vi "LVClass_WavefrontCorrector get all WFC parameter values.vi"(0 "WavefrontCorrector in":refnum<class "WavefrontCorrector.lvclass">, 11 "error in (no error)":errorcluster) -> (4 "WavefrontCorrector out":refnum<class "WavefrontCorrector.lvclass">, 6 "AllWFCParametersValues":T1[](array[typedef]), 15 "error out":errorcluster)   [LabVIEW 2020, in "WavefrontCorrector.lvclass"]
doc: "Description:\nGet current actuators positions.\n\nParameters:\nclass corrector WavefrontCorrector object adress.\nfloat position Array containing the actuators positions.\nError error_in [in] Error\nError error_out [out] Error"
uses:
  WavefrontCorrector.lvclass
  CameraParametersSetup.ctl
  CameraParameters_Type.ctl
  WavefrontCorrector.lvclass/WavefrontCorrector.ctl
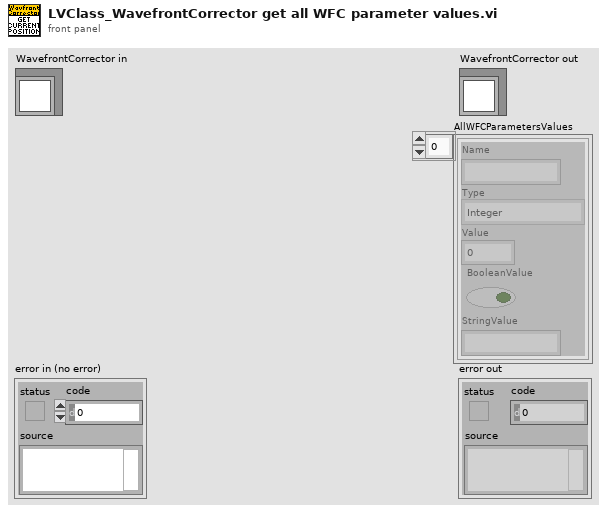
[diagram p1: front panel]
types:
  T1 = typedef "CameraParametersSetup.ctl" = cluster{"Name":string, "Type":T2, "Value":dbl, "BooleanValue":bool, "StringValue":string}
  T2 = typedef "CameraParameters_Type.ctl" = enum16{"Integer", "Real", "String", "Boolean"}
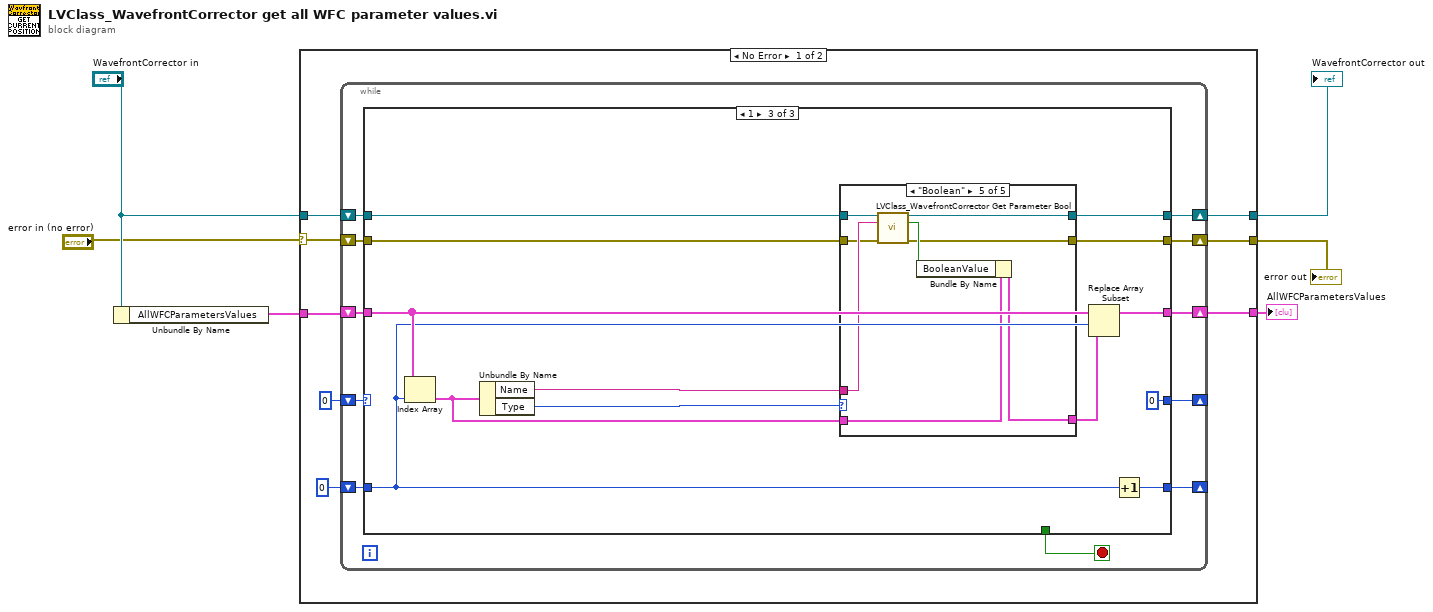
[diagram p0: block diagram]
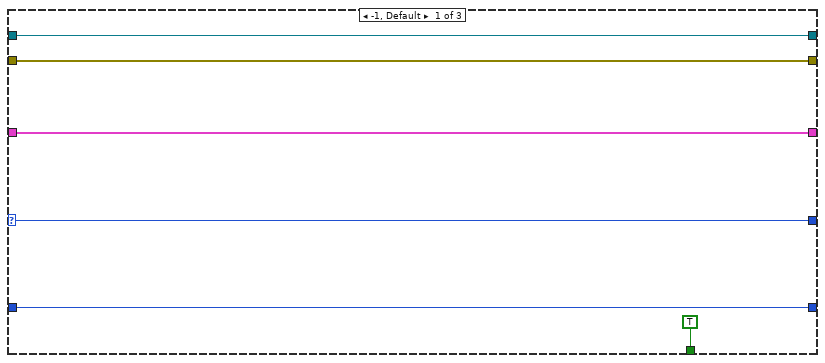
[diagram p2: hidden frame]
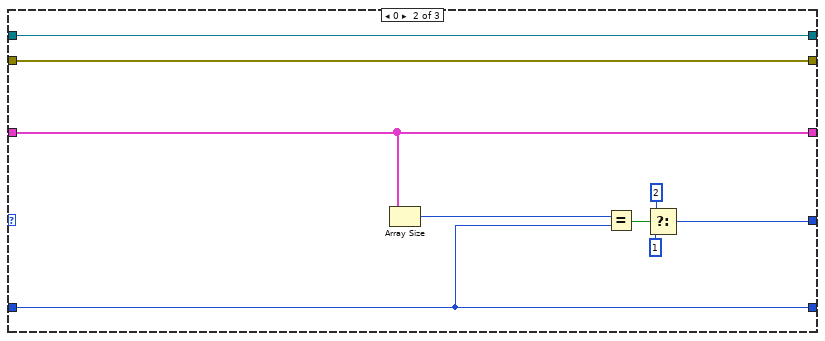
[diagram p3: hidden frame]
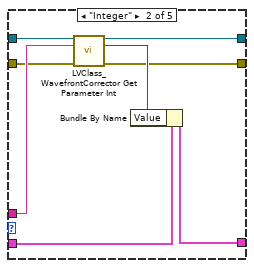
[diagram p5: hidden frame]
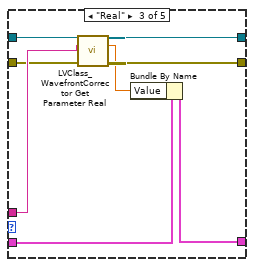
[diagram p6: hidden frame]
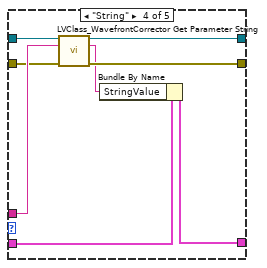
[diagram p7: hidden frame]
diagram:
  n1 = Unbundle By Name("WavefrontCorrector in") -> ("AllWFCParametersValues"=w4:T1[])
  n2 = case shown="No Error" "error in (no error)" {
    selector: "error in (no error)" -> [w10 w90]
    tunnel: [w11 w90] -> w2
    tunnel: [w12 w89] -> w5
    tunnel: "WavefrontCorrector in" -> [w14 w89]
    tunnel: [w9 _] -> w1
    tunnel: w4 -> [w7 _]
    frame No Error {
      n3 = while {
        shift-right: [w24] -> _
        shift-left: 0 -> [w23]
        shift-right: [w21] -> w11
        shift-left: w10 -> [w20]
        shift-right: [w22] -> w12
        shift-left: w14 -> [w25]
        shift-right: [w18] -> w9
        shift-left: w7 -> [w17]
        shift-right: [w15] -> _
        shift-left: 0 -> [w16]
        stop <- w19 stop-if-true
        n4 = case shown="1" w23 {
          selector: w23 -> [w26 _ _]
          tunnel: w25 -> [w30 w40 w41]
          tunnel: w20 -> [w29 w39 w42]
          tunnel: [w26 w33 0] -> w24
          tunnel: [w30 w40 w52] -> w22
          tunnel: [w29 w39 w51] -> w21
          tunnel: [TRUE _ _] -> w19
          tunnel: [w28 w38 w46] -> w18
          tunnel: w17 -> [w28 w38 w48]
          tunnel: w16 -> [w27 w36 w47]
          tunnel: [w27 w36 w50] -> w15
          frame -1, Default {
          }
          frame 0 {
            n5 = Array Size(array=w38) -> (size(s)=w37:i32)
            n6 = Equal?(x=w37, y=w36) -> (x = y?=w35:bool)
            n7 = Select(t=2, s=w35, f=1) -> (s? t:f=w33:i32)
          }
          frame 1 {
            n8 = Index Array(array=w48, index=w47) -> (element=w49:T1)
            n9 = Unbundle By Name(w49) -> ("Name"=w44:string, "Type"=w45:T2)
            n10 = case shown="\"Boolean\"" w45 {
              tunnel: w49 -> [w54 w64 w65 w73 w82]
              tunnel: [w54 w63 w66 w80 w81] -> w43
              tunnel: w44 -> [_ w62 w71 w77 w87]
              tunnel: w41 -> [w56 w61 w72 w79 w88]
              tunnel: [w56 w60 w68 w78 w85] -> w52
              tunnel: [w55 w58 w69 w75 w83] -> w51
              tunnel: w42 -> [w55 w57 w70 w76 w86]
              frame Default {
              }
              frame "Integer" {
                n11 = call "LVClass_WavefrontCorrector Get Parameter Int.vi"("WavefrontCorrector in"=w61, "parameter_name"=w62, "error in (no error)"=w57) -> ("WavefrontCorrector out"=w60:refnum<class "WavefrontCorrector.lvclass">, "value"=w59:i32, "error out"=w58:errorcluster)  [unwired: 10 in]
                n12 = Bundle By Name(cluster=w64, "Value"=w59) -> (w63:T1)
              }
              frame "Real" {
                n13 = call "LVClass_WavefrontCorrector Get Parameter Real.vi"("WavefrontCorrector in"=w72, "parameter_name"=w71, "error in (no error)"=w70) -> ("WavefrontCorrector out"=w68:refnum<class "WavefrontCorrector.lvclass">, "value"=w67:dbl, "error out"=w69:errorcluster)  [unwired: 10 in]
                n14 = Bundle By Name(cluster=w65, "Value"=w67) -> (w66:T1)
              }
              frame "String" {
                n15 = call "LVClass_WavefrontCorrector Get Parameter String.vi"("WavefrontCorrector in"=w79, "parameter_name"=w77, "error in (no error)"=w76) -> ("WavefrontCorrector out"=w78:refnum<class "WavefrontCorrector.lvclass">, "value"=w74:string, "error out"=w75:errorcluster)  [unwired: 10 in]
                n16 = Bundle By Name(cluster=w73, "StringValue"=w74) -> (w80:T1)
              }
              frame "Boolean" {
                n17 = call "LVClass_WavefrontCorrector Get Parameter Bool.vi"("WavefrontCorrector in"=w88, "parameter_name"=w87, "error in (no error)"=w86) -> ("WavefrontCorrector out"=w85:refnum<class "WavefrontCorrector.lvclass">, "value"=w84:bool, "error out"=w83:errorcluster)  [unwired: 10 in]
                n18 = Bundle By Name(cluster=w82, "BooleanValue"=w84) -> (w81:T1)
              }
            }
            n19 = Replace Array Subset(array=w48, new element=w43, index=w47) -> (w46:T1[])
            n20 = Increment(x=w47) -> (x+1=w50:i32)
          }
        }
      }
    }
    frame Error {
    }
  }
  "error out" <- w2
  "WavefrontCorrector out" <- w5
  "AllWFCParametersValues" <- w1
